vi "Read Write Text File Test.vi"(11 "Error In":errorcluster) -> (15 "Error Out":errorcluster)   [LabVIEW 2021, in "Test Files.lvlib"]
doc: "This VI has test cases for checking the functionality of Read Write Txt.vi"
uses:
  Test Files.lvlib
  <vilib>/addons/_JKI Toolkits/Caraya/classes/Test/Test.lvclass
  <vilib>/addons/_JKI Toolkits/Caraya/classes/Assert/Assert.lvclass
  CustomSortPath.lvlib
  <vilib>/addons/_JKI Toolkits/Caraya/classes/Assert/Assert Equal Value_Variant.vi
  Controls/FileOperation.ctl
panel:
  # "Read/Write To .txt File Test"
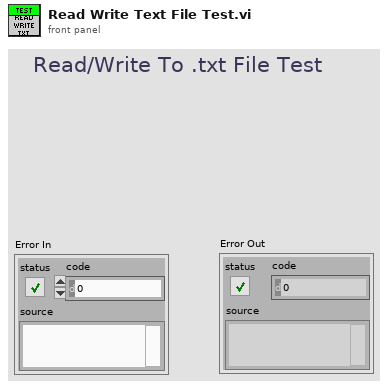
[diagram p1: front panel]
types:
  T1 = typedef "CustomSortPath.lvlib/FileOperation.ctl" = enum16{"Read", "Write"}
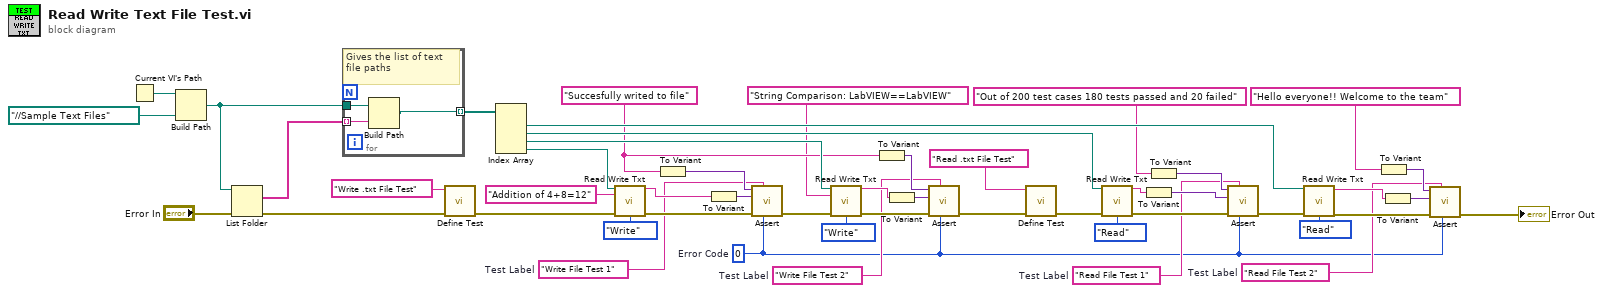
[diagram p0: block diagram]
diagram:
  w1 = 0  # Error Code
  w2 = "Read File Test 2"  # Test Label
  w3 = "Read File Test 1"  # Test Label
  w4 = "Write File Test 2"  # Test Label
  w5 = "Write File Test 1"  # Test Label
  w14 = "Succesfully writed to file"
  n1 = Current VI's Path() -> (path=w48:path)
  n2 = Build Path(base path=w48, name or relative path=path "../../Sample Text Files") -> (appended path=w43:path)
  n3 = List Folder(path=w43, error in="Error In") -> (filenames=w44:string[], error out=w45:errorcluster)  [unwired: 2 in, 2 out]
  n4 = for {
    tunnel: w44 -> [w51] mode=indexing
    tunnel: w43 -> [w52]
    tunnel: [w50] -> w42 mode=indexing
    # "Gives the list of text file paths"
    n5 = Build Path(base path=w52, name or relative path=w51) -> (appended path=w50:path)
  }
  n6 = call <vilib>:"Define Test.vi"("error in (no error)"=w45, "Label (VI Title)"="Write .txt File Test") -> ("error out"=w16:errorcluster)  [unwired: 8 in, 1 out]
  n7 = Index Array(array=w42) -> (element #1=w41:path, element #2=w34:path, element #3=w25:path, element #4=w23:path)  [unwired: 4 in]
  n8 = call "Read Write Txt.vi"("File Path"=w23, "InputString"="Addition of 4+8=12", "error in (no error)"=w16, "FileOperation"=FileOperation."Write") -> ("StringOut"=w20:string, "error out"=w17:errorcluster)  [unwired: 10 in]
  n9 = To Variant(anything=w14) -> (Variant=w22:variant)
  n10 = To Variant(anything=w20) -> (Variant=w21:variant)
  n11 = call-poly <vilib>:"Assert.vi"("error code (1)"=w1, "Label"=w5, "error in (no error)"=w17, "Y"=w21, "X"=w22) -> ("error out"=w18:errorcluster)  [unwired: 5 in, 1 out]
  n12 = call "Read Write Txt.vi"("File Path"=w25, "InputString"="String Comparison: LabVIEW==LabVIEW", "error in (no error)"=w18, "FileOperation"=FileOperation."Write") -> ("StringOut"=w12:string, "error out"=w19:errorcluster)  [unwired: 10 in]
  n13 = To Variant(anything=w14) -> (Variant=w13:variant)
  n14 = To Variant(anything=w12) -> (Variant=w11:variant)
  n15 = call-poly <vilib>:"Assert.vi"("error code (1)"=w1, "Label"=w4, "error in (no error)"=w19, "Y"=w11, "X"=w13) -> ("error out"=w10:errorcluster)  [unwired: 5 in, 1 out]
  n16 = call <vilib>:"Define Test.vi"("error in (no error)"=w10, "Label (VI Title)"="Read .txt File Test") -> ("error out"=w9:errorcluster)  [unwired: 8 in, 1 out]
  n17 = call "Read Write Txt.vi"("File Path"=w34, "error in (no error)"=w9, "FileOperation"=FileOperation."Read") -> ("StringOut"=w33:string, "error out"=w27:errorcluster)  [unwired: 11 in]
  n18 = To Variant(anything=w33) -> (Variant=w32:variant)
  n19 = To Variant(anything="Out of 200 test cases 180 tests passed and 20 failed") -> (Variant=w30:variant)
  n20 = call-poly <vilib>:"Assert.vi"("error code (1)"=w1, "Label"=w3, "error in (no error)"=w27, "Y"=w32, "X"=w30) -> ("error out"=w29:errorcluster)  [unwired: 5 in, 1 out]
  n21 = call "Read Write Txt.vi"("File Path"=w41, "error in (no error)"=w29, "FileOperation"=FileOperation."Read") -> ("StringOut"=w39:string, "error out"=w28:errorcluster)  [unwired: 11 in]
  n22 = To Variant(anything="Hello everyone!! Welcome to the team") -> (Variant=w36:variant)
  n23 = To Variant(anything=w39) -> (Variant=w38:variant)
  n24 = call-poly <vilib>:"Assert.vi"("error code (1)"=w1, "Label"=w2, "error in (no error)"=w28, "Y"=w38, "X"=w36) -> ("error out"=→"Error Out":errorcluster)  [unwired: 5 in, 1 out]
